vi "Simon main.vi"() -> ()   [LabVIEW 2020]
uses:
  Controls/State.ctl
  Controls/Simon Properties.ctl
  Simonfy/Keep Entering.ctl
  <vilib>/sound2/lvsound2.llb/Sound Output Task ID.ctl
  Controls/Simon Chars.ctl
panel:
  out "Tab Control":enum32{"Page 1", "Page 2"}(tab)
  in  "Mode choice":bool
  in  "1":bool
  in  "2":bool
  in  "3":bool
  out "Stop the Game!":bool
  out "Please choose your mode:":T1
  out "The numbe of colors you have memorized!":i32
  out "Keep Entering":T1
  in  "Please enter your answer:":T2
  out "Sequence for Player to Memorize":u32(colorbox)
  # "#todo\nclean user interface\ndifferent section"
  # "Simon"
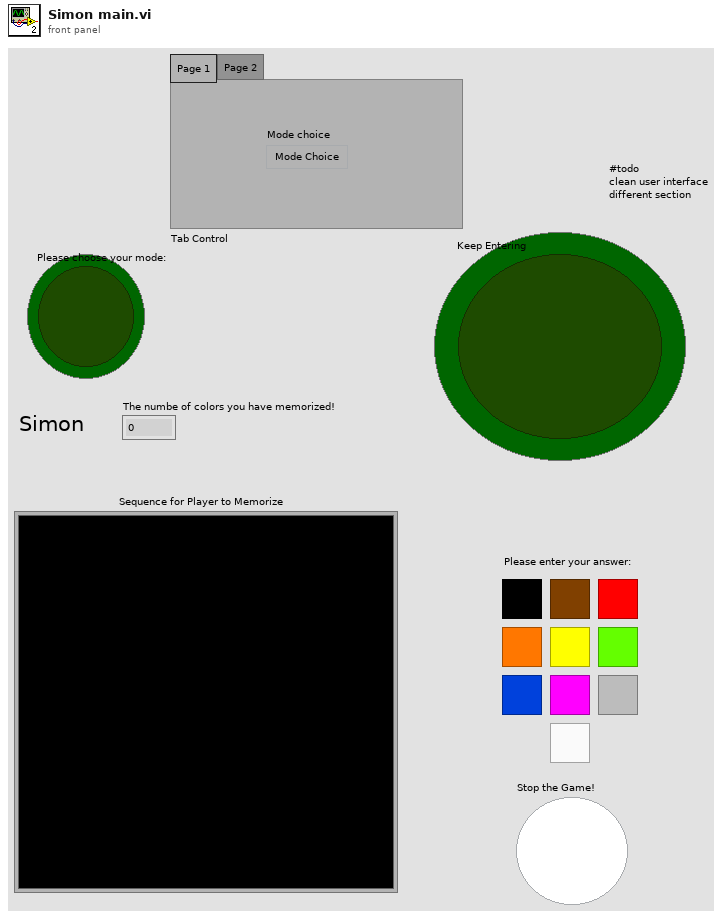
[diagram p1: front panel]
types:
  T1 = typedef "Keep Entering.ctl" = bool
  T2 = cluster{"0":bool, "7":bool, "8":bool, "9":bool, "4":bool, "5":bool, "6":bool, "1":bool, "2":bool, "3":bool}
  T3 = typedef "Sound Output Task ID.ctl" = u32
  T4 = typedef "Simon Properties.ctl" = cluster{"Sequence ":i32[], "\n Colors":u32[], "Wait Time (ms)":u32, "Last Key":i16, "Number of Key Pressed":i32, "User":bool, "Record":u32, "Username":T5}
  T5 = typedef "Simon Chars.ctl" = string
  T6 = typedef "State.ctl" = enum16{"Initialize", "Check Mode", "Add New Color", "Show Sequence", "Finsh Showing", "Wait For Event", "Check Key Press", "Success", "Fail", "Exit"}
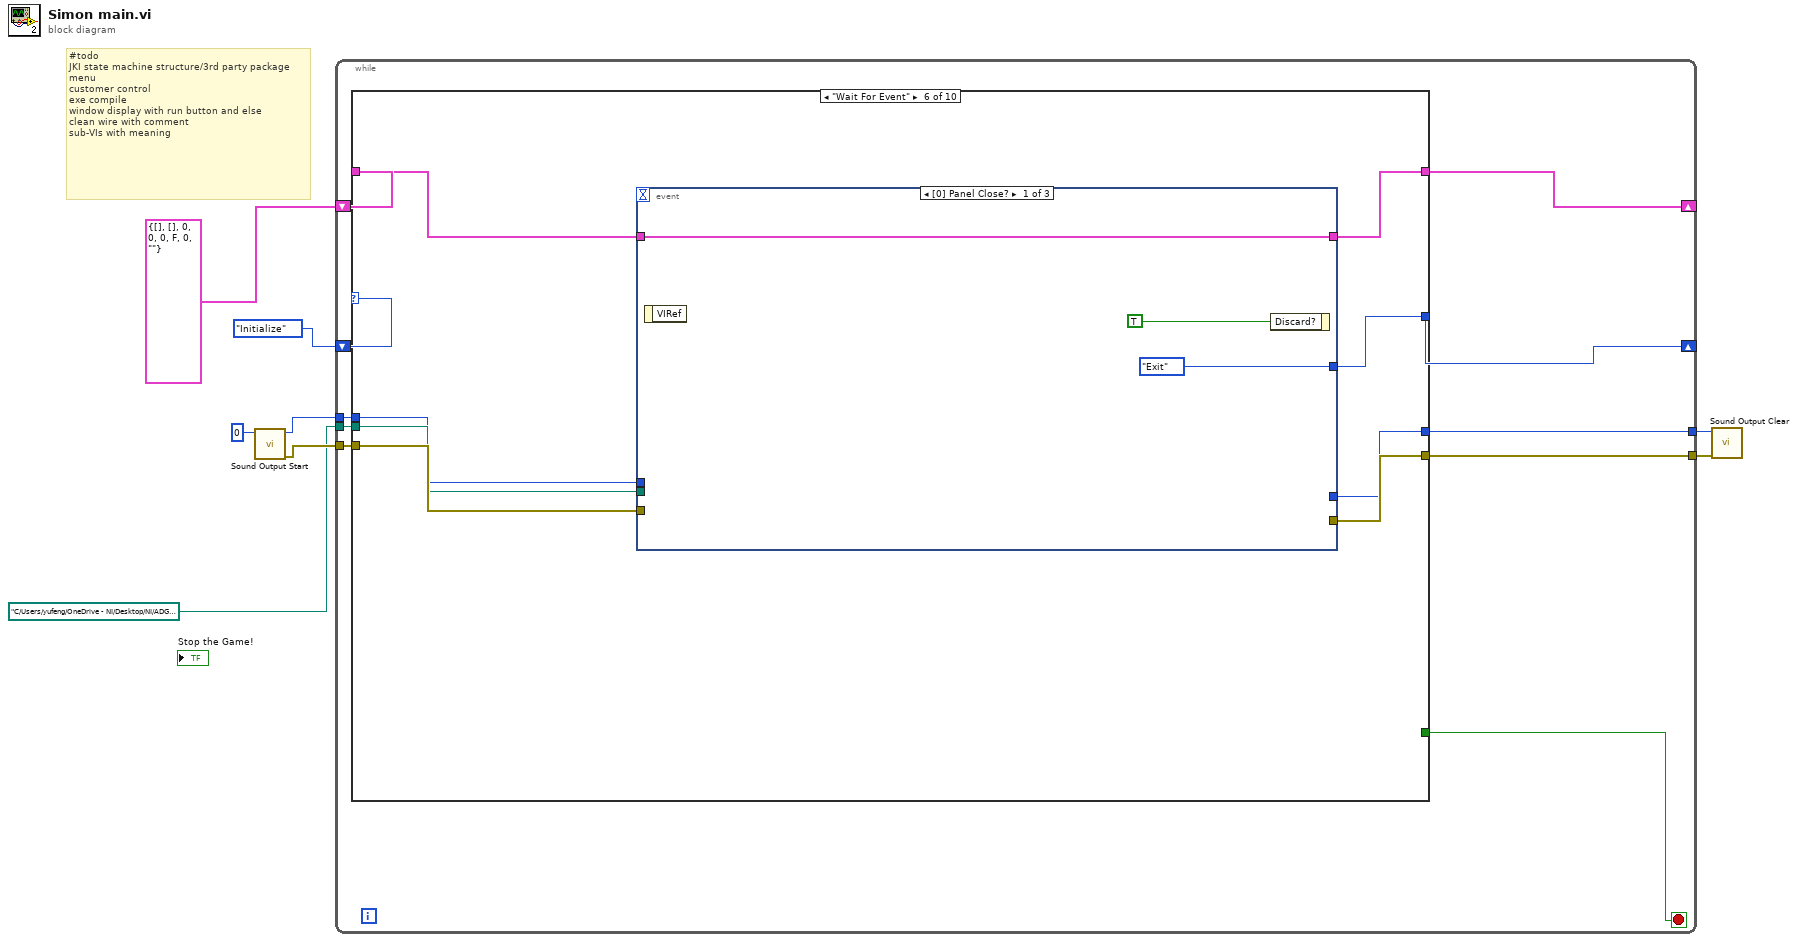
[diagram p0: block diagram]
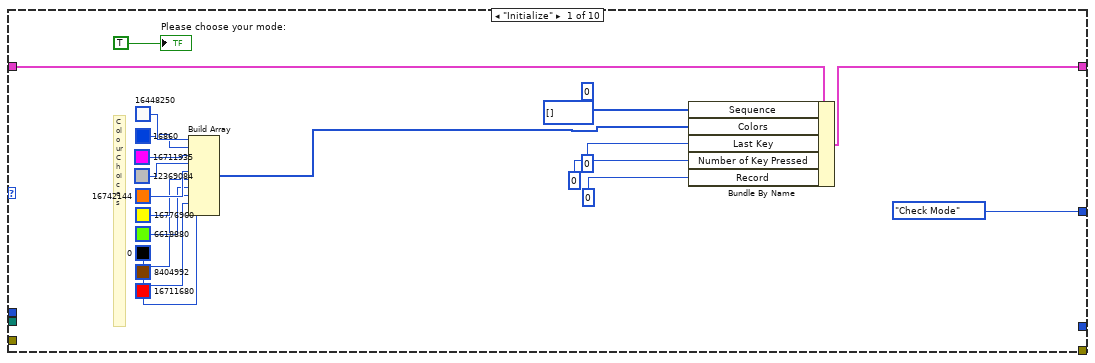
[diagram p2: hidden frame]
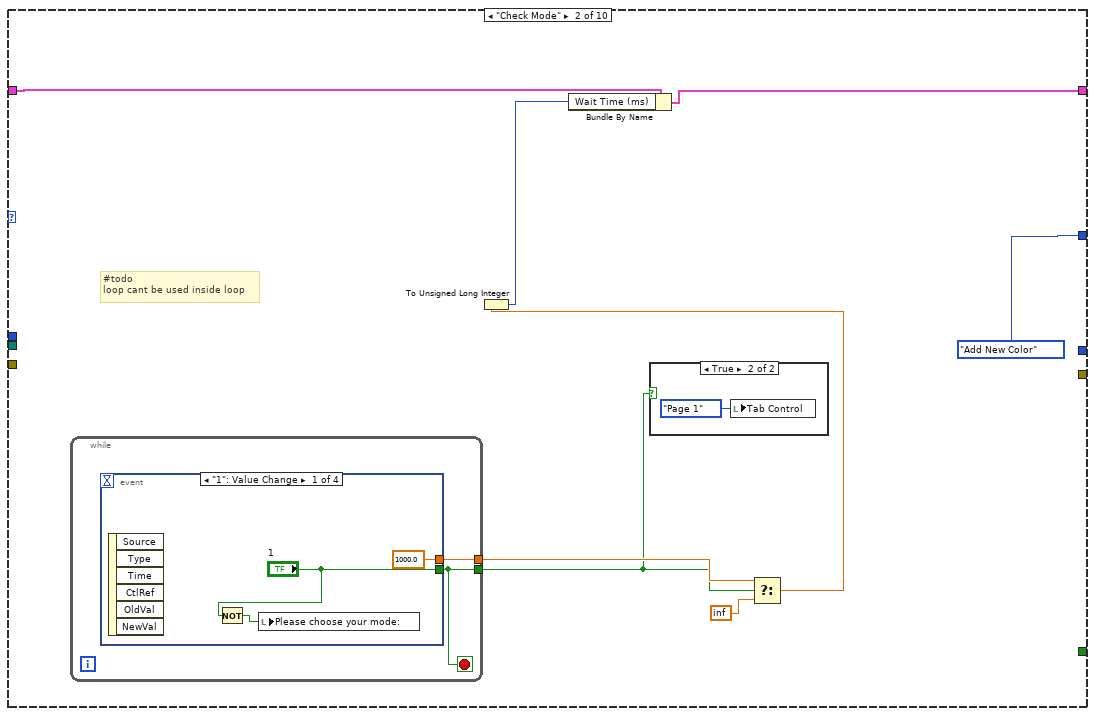
[diagram p3: hidden frame]
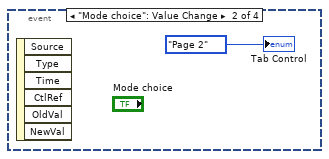
[diagram p5: hidden frame]
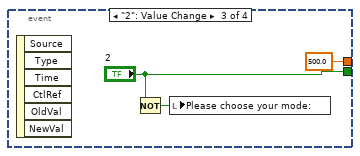
[diagram p6: hidden frame]
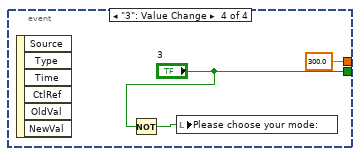
[diagram p7: hidden frame]
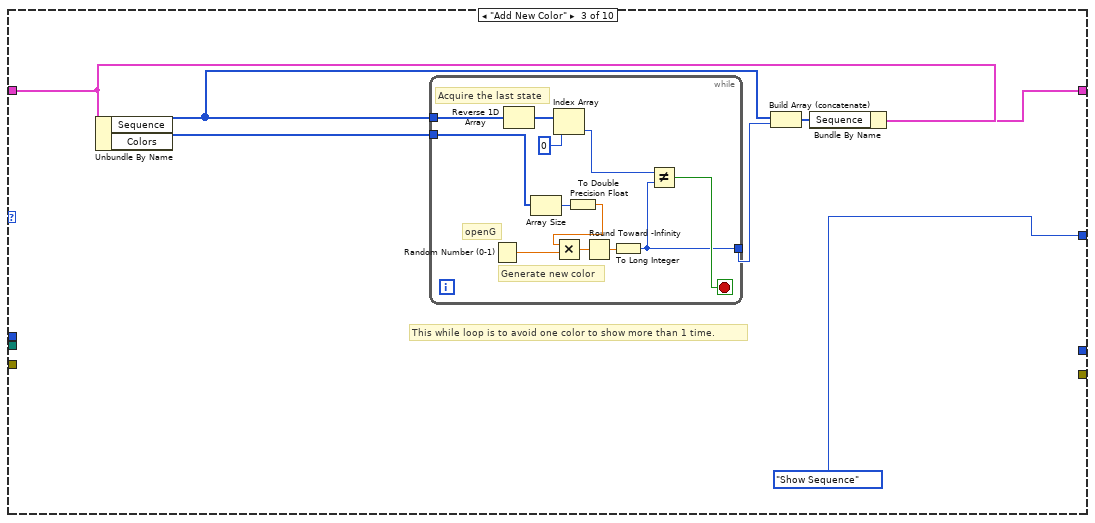
[diagram p8: hidden frame]
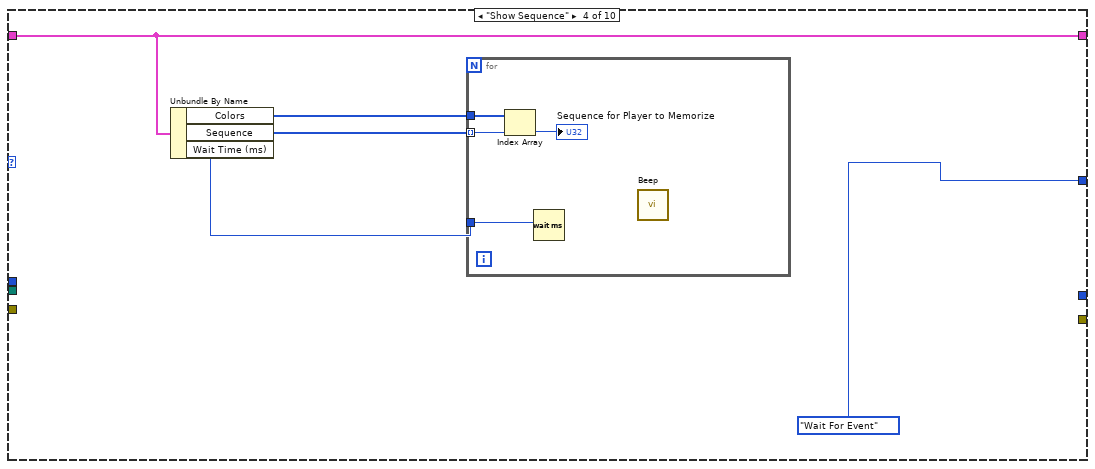
[diagram p9: hidden frame]
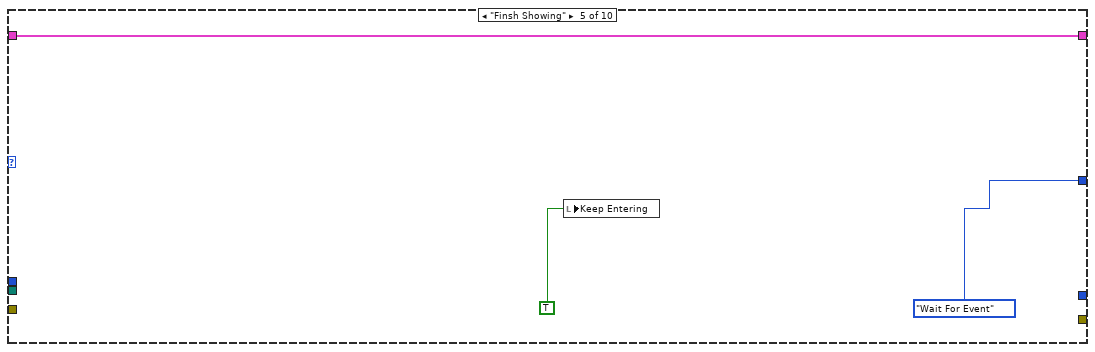
[diagram p10: hidden frame]
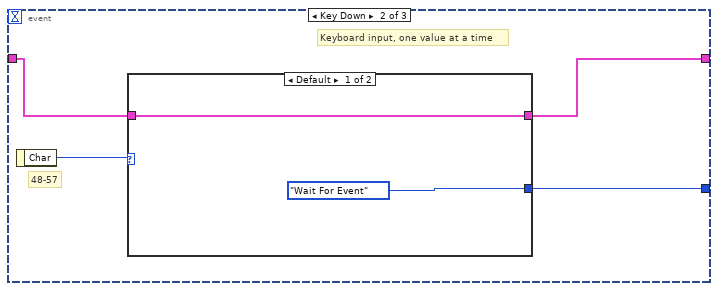
[diagram p11: hidden frame]
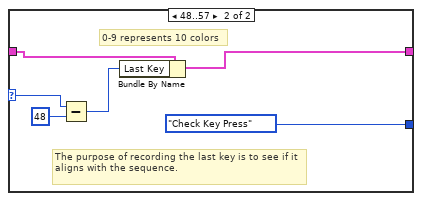
[diagram p12: hidden frame]
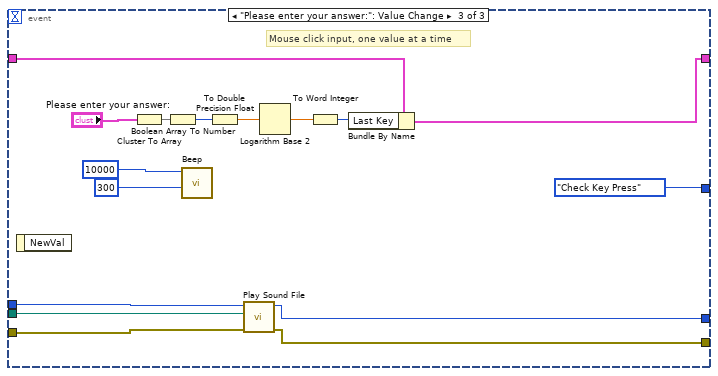
[diagram p13: hidden frame]
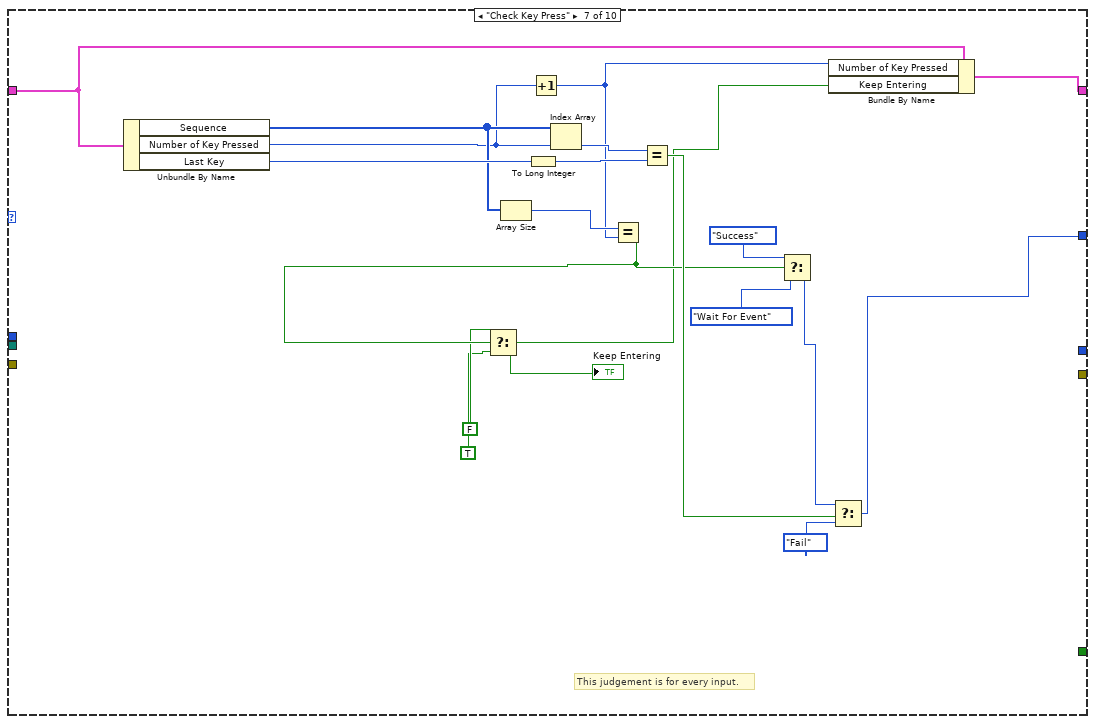
[diagram p14: hidden frame]
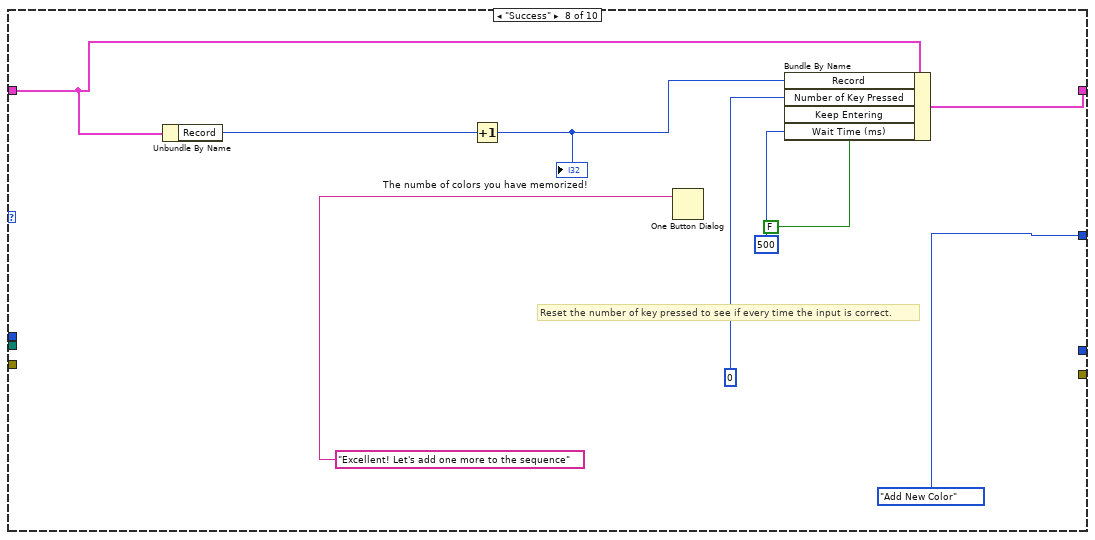
[diagram p15: hidden frame]
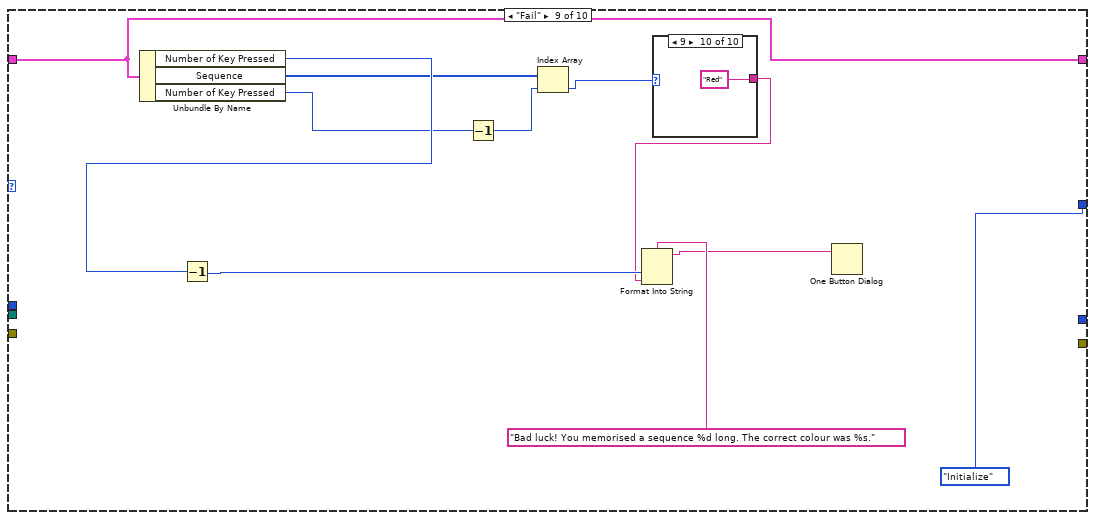
[diagram p16: hidden frame]
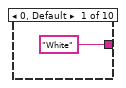
[diagram p17: hidden frame]
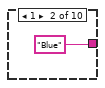
[diagram p18: hidden frame]
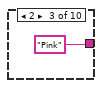
[diagram p19: hidden frame]
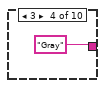
[diagram p20: hidden frame]
diagram:
  # "#todo\nJKI state machine structure/3rd party package\nmenu\ncustomer control\nexe compile\nwindow display with run button and else\nclean wire with comment\nsub-VIs with meaning"
  n1 = call <vilib>:"Sound Output Start.vi"("task ID"=T3 0) -> ("error out"=w5:errorcluster, "task ID out"=w1:T3)  [unwired: 9 in]
  n2 = while {
    shift-right: [w15] -> _
    shift-left: T4 {"Sequence "=[], "\n Colors"=[], "Wait Time (ms)"=0, "Last Key"=0, "Number of Key Pressed"=0, "User"=FALSE, "Record"=0, "Username"=""} -> [w16]
    shift-right: [w14] -> _
    shift-left: State."Initialize" -> [w18]
    tunnel: w5 -> [w13]
    tunnel: path "C:/Users/yufeng/OneDrive - NI/Desktop/NI/ADG CCS AE/Simon/MyRepository/311594Preview.wav" ("path") -> [w12]
    tunnel: [w11] -> w3
    tunnel: [w10] -> w2
    tunnel: w1 -> [w9]
    stop <- w17 stop-if-true
    n3 = case shown="\"Wait For Event\"" w18 {
      tunnel: [_ _ _ _ _ _ _ _ _ TRUE] -> w17
      tunnel: w16 -> [w20 w41 w61 w82 w89 w97 w144 w154 w162 w179]
      tunnel: [w33 w39 w60 w82 w89 w96 w143 w153 w162 w179] -> w15
      tunnel: [State."Check Mode" State."Add New Color" State."Show Sequence" State."Wait For Event" State."Wait For Event" w95 w141 State."Add New Color" State."Initialize" State."Exit"] -> w14
      tunnel: w13 -> [_ _ _ _ _ w94 _ _ _ _]
      tunnel: w12 -> [_ _ _ _ _ w93 _ _ _ _]
      tunnel: [_ _ _ _ _ w92 _ _ _ _] -> w11
      tunnel: [_ _ _ _ _ w91 _ _ _ _] -> w10
      tunnel: w9 -> [_ _ _ _ _ w90 _ _ _ _]
      frame "Initialize" {
        (unwired) 0 ("Wait Time (ms)")
        # "Colour Choices"
        n4 = Build Array(u32 16448250 ("Color Box"), u32 16860 ("Color Box"), u32 16711935 ("Color Box"), u32 12369084 ("Color Box"), u32 16742144 ("Color Box"), u32 16776960 ("Color Box"), u32 6618880 ("Color Box"), u32 0 ("Color Box"), u32 8404992 ("Color Box"), u32 16711680 ("Color Box")) -> (w21:u32[])
        n5 = Bundle By Name(cluster=w20, "Sequence"=i32[] [], "Colors"=w21, "Last Key"=i16 0, "Number of Key Pressed"=0 ("Nmber of Key Pressed"), "Record"=0 ("Tally")) -> (w33:T4)
        "Please choose your mode:" <- T1 TRUE ("Please choose your mode:")
      }
      frame "Check Mode" {
        # "#todo\nloop cant be used inside loop"
        n6 = while {
          tunnel: [w47] -> w42
          tunnel: [w48] -> w43
          stop <- w47 stop-if-true
          n7 = event shown="[0] \"1\": Value Change" {
            selector: _ -> [_ _ _ _]
            dyn-events: _ -> [_ _ _ _]
            timeout: _ -> [_ _ _ _]
            tunnel: ["1" _ "2" "3"] -> w47
            tunnel: [1000.0 ("t") _ 500.0 ("t") 300.0 ("t")] -> w48
            event "1": Value Change {
              n8 = event-data() -> ()  [unwired: 1 in, 6 out]
              n9 = Not(x="1") -> (.not. x?=w50:bool)
              n10 = local write "Please choose your mode:"(w50) -> ()
            }
            event "Mode choice": Value Change {
              n11 = event-data() -> ()  [unwired: 1 in, 6 out]
              "Tab Control" <- enum32{"Page 1", "Page 2"}."Page 2" ("Tab Control")
            }
            event "2": Value Change {
              n12 = event-data() -> ()  [unwired: 1 in, 6 out]
              n13 = Not(x="2") -> (.not. x?=w53:bool)
              n14 = local write "Please choose your mode:"(w53) -> ()
            }
            event "3": Value Change {
              n15 = event-data() -> ()  [unwired: 1 in, 6 out]
              n16 = Not(x="3") -> (.not. x?=w56:bool)
              n17 = local write "Please choose your mode:"(w56) -> ()
            }
          }
        }
        n18 = case shown="True" w42 {
          frame False {
          }
          frame True {
            n19 = local write "Tab Control"(enum32{"Page 1", "Page 2"}."Page 1" ("Tab Control")) -> ()
          }
        }
        n20 = Select(t=w43, s=w42, f=inf) -> (s? t:f=w45:dbl)
        n21 = To Unsigned Long Integer(number=w45) -> (unsigned 32bit integer=w40:u32)
        n22 = Bundle By Name(cluster=w41, "Wait Time (ms)"=w40) -> (w39:T4)
      }
      frame "Add New Color" {
        # "This while loop is to avoid one color to show more than 1 time."
        n23 = Unbundle By Name(w61) -> ("Sequence"=w64:i32[], "Colors"=w65:u32[])
        n24 = while {
          tunnel: w64 -> [w77]
          tunnel: w65 -> [w74]
          tunnel: [w66] -> w63
          stop <- w67 stop-if-true
          # "openG"
          # "Generate new color"
          # "Acquire the last state"
          n25 = Random Number (0-1)() -> (number: 0 to 1=w73:dbl)
          n26 = Reverse 1D Array(array=w77) -> (reversed array=w76:i32[])
          n27 = Array Size(array=w74) -> (size(s)=w71:i32)
          n28 = Index Array(array=w76, index=0) -> (element=w68:i32)
          n29 = To Double Precision Float(number=w71) -> (double precision float=w70:dbl)
          n30 = Multiply(x=w70, y=w73) -> (x*y=w72:dbl)
          n31 = Round Toward -Infinity(1:w72) -> (0:w69:dbl)
          n32 = To Long Integer(number=w69) -> (32bit integer=w66:i32)
          n33 = Not Equal?(x=w68, y=w66) -> (x != y?=w67:bool)
        }
        n34 = Build Array (concatenate)(w64, w63) -> (w62:i32[])
        n35 = Bundle By Name(cluster=w61, "Sequence"=w62) -> (w60:T4)
      }
      frame "Show Sequence" {
        n36 = Unbundle By Name(w82) -> ("Colors"=w81:u32[], "Sequence"=w80:i32[], "Wait Time (ms)"=w79:u32)
        n37 = for {
          tunnel: w81 -> [w86]
          tunnel: w80 -> [w85] mode=indexing
          tunnel: w79 -> [w83]
          n38 = Index Array(array=w86, index=w85) -> (element=→"Sequence for Player to Memorize":u32)
          n39 = Wait (ms)(milliseconds to wait=w83) -> ()  [unwired: 1 out]
          n40 = call <vilib>:"Beep.vi"() -> ()  [unwired: 12 in]
        }
      }
      frame "Finsh Showing" {
        n41 = local write "Keep Entering"(T1 TRUE ("Keep Entering")) -> ()
      }
      frame "Wait For Event" {
        n42 = event shown="[0] Panel Close?" {
          selector: _ -> [_ _ _]
          dyn-events: _ -> [_ _ _]
          timeout: _ -> [_ _ _]
          tunnel: w97 -> [w100 w103 w120]
          tunnel: [w100 w102 w121] -> w96
          tunnel: [State."Exit" w101 State."Check Key Press"] -> w95
          tunnel: w94 -> [_ _ w117]
          tunnel: w93 -> [_ _ w116]
          tunnel: [_ _ w115] -> w92
          tunnel: [_ _ w114] -> w91
          tunnel: w90 -> [_ _ w113]
          event Panel Close? {
            n43 = event-data() -> ()  [unwired: 1 in, 1 out]
            n44 = event-data("Discard?"=TRUE) -> ()  [unwired: 1 in, 1 out]
          }
          event Key Down {
            # "Keyboard input, one value at a time"
            # "48-57"
            n45 = event-data() -> ("Char"=w104:i16)  [unwired: 1 in]
            n46 = case shown="Default" w104 {
              selector: w104 -> [_ w110]
              tunnel: w103 -> [w106 w112]
              tunnel: [w106 w111] -> w102
              tunnel: [State."Wait For Event" State."Check Key Press"] -> w101
              frame Default {
              }
              frame 48..57 {
                # "The purpose of recording the last key is to see if it aligns with the sequence."
                # "0-9 represents 10 colors"
                n47 = Subtract(x=w110, y=i16 48) -> (x-y=w108:i16)
                n48 = Bundle By Name(cluster=w112, "Last Key"=w108) -> (w111:T4)
              }
            }
          }
          event "Please enter your answer:": Value Change {
            # "Mouse click input, one value at a time"
            n49 = event-data() -> ()  [unwired: 1 in, 1 out]
            n50 = Cluster To Array(cluster="Please enter your answer:") -> (array=w127:bool[])
            n51 = Boolean Array To Number(Boolean array=w127) -> (number=w126:u32)
            n52 = call <vilib>:"Beep.vi"("duration (msec)"=u32 300, "frequency (Hz)"=u32 10000) -> ()  [unwired: 10 in]
            n53 = To Double Precision Float(number=w126) -> (double precision float=w125:dbl)
            n54 = call <vilib>:"Play Sound File.vi"("error in (no error)"=w117, "path"=w116, "device ID"=w113) -> ("error out"=w115:errorcluster, "task ID"=w114:T3)  [unwired: 7 in]
            n55 = Logarithm Base 2(1:w125) -> (0:w124:dbl)
            n56 = To Word Integer(number=w124) -> (16bit integer=w123:i16)
            n57 = Bundle By Name(cluster=w120, "Last Key"=w123) -> (w121:T4)
          }
        }
      }
      frame "Check Key Press" {
        # "This judgement is for every input."
        n58 = Unbundle By Name(w144) -> ("Sequence"=w140:i32[], "Number of Key Pressed"=w134:i32, "Last Key"=w145:i16)
        n59 = Array Size(array=w140) -> (size(s)=w139:i32)
        n60 = To Long Integer(number=w145) -> (32bit integer=w146:i32)
        n61 = Increment(x=w134) -> (x+1=w133:i32)
        n62 = Index Array(array=w140, index=w134) -> (element=w147:i32)
        n63 = Equal?(x=w139, y=w133) -> (x = y?=w132:bool)
        n64 = Select(t=FALSE, s=w132, f=TRUE) -> (s? t:f=w129:bool)
        "Keep Entering" <- w129
        n65 = Equal?(x=w147, y=w146) -> (x = y?=w138:bool)
        n66 = Select(t=State."Success", s=w132, f=State."Wait For Event") -> (s? t:f=w135:T6)
        n67 = Bundle By Name(cluster=w144, "Number of Key Pressed"=w133, "Keep Entering"=w129) -> (w143:T4)
        n68 = Select(t=w135, s=w138, f=State."Fail") -> (s? t:f=w141:T6)
      }
      frame "Success" {
        # "Reset the number of key pressed to see if every time the input is correct."
        n69 = Unbundle By Name(w154) -> ("Record"=w156:u32)
        n70 = Increment(x=w156) -> (x+1=w155:u32)
        "The numbe of colors you have memorized!" <- w155
        n71 = One Button Dialog(message="Excellent! Let's add one more to the sequence") -> ()  [unwired: 1 in, 1 out]
        n72 = Bundle By Name(cluster=w154, "Record"=w155, "Number of Key Pressed"=0, "Keep Entering"=FALSE, "Wait Time (ms)"=u32 500) -> (w153:T4)
      }
      frame "Fail" {
        n73 = Unbundle By Name(w162) -> ("Number of Key Pressed"=w166:i32, "Sequence"=w161:i32[], "Number of Key Pressed"=w158:i32)
        n74 = Decrement(x=w166) -> (x-1=w165:i32)
        n75 = Decrement(x=w158) -> (x-1=w157:i32)
        n76 = Index Array(array=w161, index=w157) -> (element=w160:i32)
        n77 = case shown="9" w160 {
          tunnel: ["White" "Blue" "Pink" "Gray" "Orange" "Yellow" "GREEN" "Black" "Brown" "Red"] -> w159
          frame 0, Default {
          }
          frame 1 {
          }
          frame 2 {
          }
          frame 3 {
          }
          frame 4 {
          }
          frame 5 {
          }
          frame 6 {
          }
          frame 7 {
          }
          frame 8 {
          }
          frame 9 {
          }
        }
        n78 = Format Into String(format string="Bad luck! You memorised a sequence %d long. The correct colour was %s." ("message"), w165, w159) -> (resulting string=w164:string)  [unwired: 2 in, 1 out]
        n79 = One Button Dialog(message=w164) -> ()  [unwired: 1 in, 1 out]
      }
      frame "Exit", Default {
      }
    }
  }
  n80 = call <vilib>:"Sound Output Clear.vi"("error in (no error)"=w3, "task ID"=w2) -> ()  [unwired: 9 in, 1 out]
